vi "Serial.vi"(2 "PortName":string, 12 "Run":bool, 14 "Calibration":bool) -> (0 "DS18b20":string, 4 "DS18b20":dbl[unit][](array[numeric]), 5 "SHT11":string, 6 "MPX":dbl[](array[numeric]), 7 "MPXV7002":string, 8 "EEP":dbl[](array[numeric]), 9 "EEP":string, 10 "SHT/H":dbl[unit][](array[numeric]), 11 "Complete":bool, 15 "SHT/T":dbl[](array[numeric]))   [LabVIEW 2018]
panel:
  out "eep":bool
  out "mpxv":bool
  out "sht":bool
  out "ds":bool
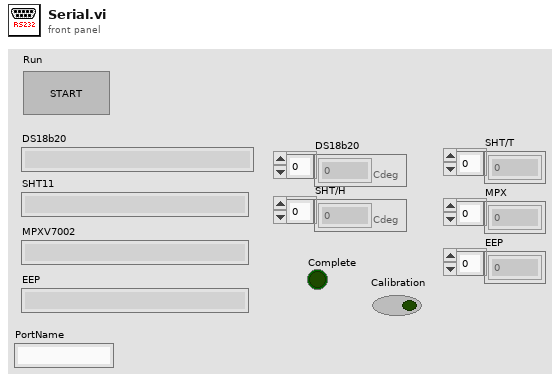
[diagram p1: front panel]
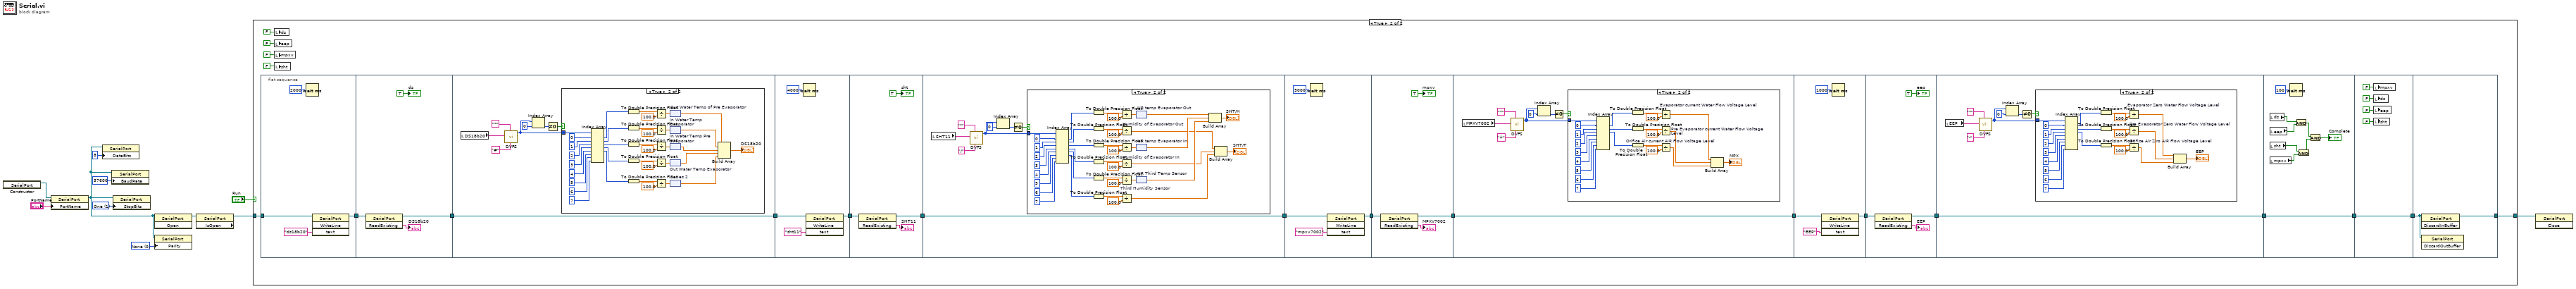
[diagram p0: block diagram]
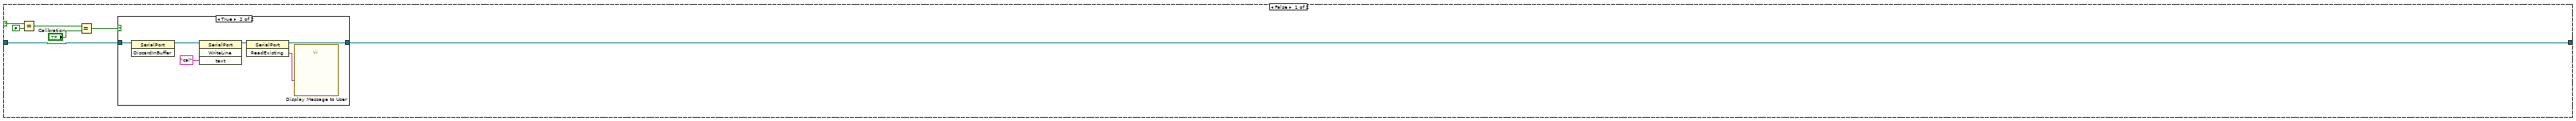
[diagram p2: hidden frame]
diagram:
  w7 = 1 items=["None", "One", "Two", "OnePointFive"] ("StopBits")
  w6 = 0 items=["None", "Odd", "Even", "Mark", "Space"] ("Parity")
  n1 = constructor class="SerialPort"() -> (reference out=w2:refnum<k24>)  [unwired: 3 in, 2 out]
  n2 = property class="SerialPort"(reference=w2, "PortName"="PortName") -> (reference out=w4:refnum<k24>)  [unwired: 1 in, 1 out]
  n3 = property class="SerialPort"(reference=w4, "DataBits"=8) -> ()  [unwired: 1 in, 2 out]
  n4 = property class="SerialPort"(reference=w4, "BaudRate"=57600) -> ()  [unwired: 1 in, 2 out]
  n5 = property class="SerialPort"(reference=w4, "StopBits"=w7) -> ()  [unwired: 1 in, 2 out]
  n6 = invoke class="SerialPort" method="Open"(reference=w4) -> (reference out=w9:refnum<k24>)  [unwired: 2 in, 2 out]
  n7 = property class="SerialPort"(reference=w4, "Parity"=w6) -> ()  [unwired: 1 in, 2 out]
  n8 = property class="SerialPort" props=["IsOpen"](reference=w9) -> (reference out=w3:refnum<k24>)  [unwired: 1 in, 2 out]
  n9 = case shown="True" "Run" {
    selector: "Run" -> [w17 _]
    tunnel: w3 -> [w18 w28]
    tunnel: [w12 w27] -> w11
    frame False {
      n10 = Equal?(x=w17, y=FALSE) -> (x = y?=w15:bool)
      n11 = Equal?(x=w15, y="Calibration") -> (x = y?=w13:bool)
      n12 = case shown="True" w13 {
        tunnel: w18 -> [w19 w21]
        tunnel: [w19 w24] -> w12
        frame False {
        }
        frame True {
          n13 = invoke class="SerialPort" method="DiscardInBuffer"(reference=w21) -> (reference out=w20:refnum<k24>)  [unwired: 2 in, 2 out]
          n14 = invoke class="SerialPort" method="WriteLine"(reference=w20, "text"="cal" ("write buffer")) -> (reference out=w25:refnum<k24>)  [unwired: 2 in, 3 out]
          n15 = invoke class="SerialPort" method="ReadExisting"(reference=w25) -> (reference out=w24:refnum<k24>, "ReadExisting"=w22:string)  [unwired: 2 in, 1 out]
          n16 = call "Display Message to User"("Message"=w22) -> ()  [unwired: 9 in, 2 out]
        }
      }
    }
    frame True {
      n17 = flat-sequence {
        tunnel: [w47] -> w45
        tunnel: w28 -> [w46]
        tunnel: w45 -> [w53]
        tunnel: [w52] -> w44
        tunnel: w44 -> [w61]
        tunnel: [w61] -> w43
        tunnel: w43 -> [w100]
        tunnel: [w97] -> w42
        tunnel: w42 -> [w103]
        tunnel: [w102] -> w41
        tunnel: w41 -> [w112]
        tunnel: [w112] -> w40
        tunnel: w40 -> [w152]
        tunnel: [w151] -> w39
        tunnel: w39 -> [w158]
        tunnel: [w156] -> w38
        tunnel: w38 -> [w166]
        tunnel: [w166] -> w37
        tunnel: w37 -> [w192]
        tunnel: [w189] -> w36
        tunnel: w36 -> [w195]
        tunnel: [w194] -> w35
        tunnel: w35 -> [w204]
        tunnel: [w204] -> w34
        tunnel: [w234] -> w33
        tunnel: w34 -> [w234]
        tunnel: w33 -> [w240]
        tunnel: [w240] -> w32
        tunnel: w32 -> [w242]
        tunnel: [w241] -> w27
        frame #0 {
          n18 = Wait (ms)(milliseconds to wait=u32 2000) -> ()  [unwired: 1 out]
          n19 = invoke class="SerialPort" method="WriteLine"(reference=w46, "text"="ds18b20") -> (reference out=w47:refnum<k24>)  [unwired: 2 in, 3 out]
        }
        frame #1 {
          n20 = invoke class="SerialPort" method="ReadExisting"(reference=w53) -> (reference out=w52:refnum<k24>, "ReadExisting"=→"DS18b20":string)  [unwired: 2 in, 1 out]
          "ds" <- TRUE ("DS")
        }
        frame #2 {
          n21 = local read "DS18b20"() -> (w55:string)
          n22 = call "DVFS.vi"("Start string"="*", "string"=w55, "end string"="#") -> ("Output"=w54:i32[])  [unwired: 3 in, 2 out]
          n23 = Index Array(array=w54, index=0) -> (element=w57:i32)
          n24 = Not Equal To 0?(x=w57) -> (x != 0?=w56:bool)
          n25 = case shown="True" w56 {
            tunnel: w54 -> [_ w96]
            frame False {
            }
            frame True {
              n26 = Index Array(array=w96, index #1=0 ("index"), index #2=1 ("index"), index #3=2 ("index"), index #4=3 ("index"), index #5=4 ("index"), index #6=5 ("index"), index #7=6 ("index"), index #8=7 ("index")) -> (element #1=w72:i32, element #2=w71:i32, element #3=w70:i32, element #4=w69:i32, element #5=w68:i32)  [unwired: 3 out]
              n27 = To Double Precision Float(number=w72) -> (double precision float=w87:dbl)
              n28 = To Double Precision Float(number=w71) -> (double precision float=w83:dbl)
              n29 = To Double Precision Float(number=w70) -> (double precision float=w81:dbl)
              n30 = To Double Precision Float(number=w69) -> (double precision float=w79:dbl)
              n31 = To Double Precision Float(number=w68) -> (double precision float=w75:dbl)
              n32 = Divide(x=w87, y=100.0) -> (x/y=w85:dbl)
              n33 = Divide(x=w83, y=100.0) -> (x/y=w84:dbl)
              n34 = Divide(x=w81, y=100.0) -> (x/y=w77:dbl)
              n35 = Divide(x=w79, y=100.0) -> (x/y=w76:dbl)
              n36 = Divide(x=w75, y=100.0) -> (x/y=w73:dbl)
              n37 = node "Out Water Temp of Pre Evaporator"(w85) -> (w67:dbl[unit])
              n38 = node "In Water Temp Evaporator"(w84) -> (w66:dbl[unit])
              n39 = node "In Water Temp Pre Evaporator"(w77) -> (w65:dbl[unit])
              n40 = node "Out Water Temp Evaporator"(w76) -> (w64:dbl[unit])
              n41 = node "Series 2"(w73) -> (w63:dbl[unit])
              n42 = Build Array(w67, w66, w65, w64, w63) -> (→"DS18b20":dbl[unit][])
            }
          }
        }
        frame #3 {
          n43 = Wait (ms)(milliseconds to wait=u32 4000) -> ()  [unwired: 1 out]
          n44 = invoke class="SerialPort" method="WriteLine"(reference=w100, "text"="sht11" ("write buffer")) -> (reference out=w97:refnum<k24>)  [unwired: 2 in, 3 out]
        }
        frame #4 {
          n45 = invoke class="SerialPort" method="ReadExisting"(reference=w103) -> (reference out=w102:refnum<k24>, "ReadExisting"=→"SHT11":string)  [unwired: 2 in, 1 out]
          "sht" <- TRUE ("SHT")
        }
        frame #5 {
          n46 = local read "SHT11"() -> (w106:string)
          n47 = call "DVFS.vi"("Start string"="*", "string"=w106, "end string"="/") -> ("Output"=w105:i32[])  [unwired: 3 in, 2 out]
          n48 = Index Array(array=w105, index=0) -> (element=w108:i32)
          n49 = Not Equal To 0?(x=w108) -> (x != 0?=w107:bool)
          n50 = case shown="True" w107 {
            tunnel: w105 -> [_ w150]
            frame False {
            }
            frame True {
              n51 = Index Array(array=w150, index #1=0 ("index"), index #2=1 ("index"), index #3=2 ("index"), index #4=3 ("index"), index #5=4 ("index"), index #6=5 ("index"), index #7=6 ("index"), index #8=7 ("index")) -> (element #1=w126:i32, element #2=w125:i32, element #3=w124:i32, element #4=w123:i32, element #5=w122:i32, element #6=w121:i32)  [unwired: 2 out]
              n52 = To Double Precision Float(number=w126) -> (double precision float=w141:dbl)
              n53 = To Double Precision Float(number=w125) -> (double precision float=w132:dbl)
              n54 = To Double Precision Float(number=w124) -> (double precision float=w139:dbl)
              n55 = To Double Precision Float(number=w123) -> (double precision float=w130:dbl)
              n56 = To Double Precision Float(number=w122) -> (double precision float=w137:dbl)
              n57 = To Double Precision Float(number=w121) -> (double precision float=w128:dbl)
              n58 = Divide(x=w141, y=100.0) -> (x/y=w135:dbl)
              n59 = Divide "Humidity of Evaporator Out"(x=w132, y=100.0) -> (x/y=w117:dbl)
              n60 = Divide(x=w139, y=100.0) -> (x/y=w134:dbl)
              n61 = Divide "Humidity of Evaporator In"(x=w130, y=100.0) -> (x/y=w116:dbl)
              n62 = Divide(x=w137, y=100.0) -> (x/y=w133:dbl)
              n63 = Divide "Third Humidity Sensor"(x=w128, y=100.0) -> (x/y=w115:dbl)
              n64 = node "AIR temp Evaporator Out"(w135) -> (w120:dbl[unit])
              n65 = node "AIR temp Evaporator In"(w134) -> (w119:dbl[unit])
              n66 = node "AIR Third Temp Sensor"(w133) -> (w118:dbl[unit])
              n67 = Build Array(w120, w119, w118) -> (→"SHT/H":dbl[unit][])
              n68 = Build Array(w117, w116, w115) -> (→"SHT/T":dbl[])
            }
          }
        }
        frame #6 {
          n69 = Wait (ms)(milliseconds to wait=u32 5000) -> ()  [unwired: 1 out]
          n70 = invoke class="SerialPort" method="WriteLine"(reference=w152, "text"="mpxv7002" ("write buffer")) -> (reference out=w151:refnum<k24>)  [unwired: 2 in, 3 out]
        }
        frame #7 {
          n71 = invoke class="SerialPort" method="ReadExisting"(reference=w158) -> (reference out=w156:refnum<k24>, "ReadExisting"=→"MPXV7002":string)  [unwired: 2 in, 1 out]
          "mpxv" <- TRUE ("MPXV")
        }
        frame #8 {
          n72 = local read "MPXV7002"() -> (w160:string)
          n73 = call "DVFS.vi"("Start string"="*", "string"=w160, "end string"="+") -> ("Output"=w159:i32[])  [unwired: 3 in, 2 out]
          n74 = Index Array(array=w159, index=0) -> (element=w162:i32)
          n75 = Not Equal To 0?(x=w162) -> (x != 0?=w161:bool)
          n76 = case shown="True" w161 {
            tunnel: w159 -> [_ w188]
            frame False {
            }
            frame True {
              n77 = Index Array(array=w188, index #1=0 ("index"), index #2=1 ("index"), index #3=2 ("index"), index #4=3 ("index"), index #5=4 ("index"), index #6=5 ("index"), index #7=6 ("index"), index #8=7 ("index")) -> (element #1=w173:i32, element #2=w172:i32, element #3=w171:i32)  [unwired: 5 out]
              n78 = To Double Precision Float(number=w173) -> (double precision float=w179:dbl)
              n79 = To Double Precision Float(number=w172) -> (double precision float=w177:dbl)
              n80 = To Double Precision Float(number=w171) -> (double precision float=w175:dbl)
              n81 = Divide "Evaporator current Water Flow Voltage Level"(x=w179, y=100.0) -> (x/y=w170:dbl)
              n82 = Divide "Pre Evaporator current Water Flow Voltage Level"(x=w177, y=100.0) -> (x/y=w169:dbl)
              n83 = Divide "Orifice Air current AIR Flow Voltage Level"(x=w175, y=100.0) -> (x/y=w168:dbl)
              n84 = Build Array(w170, w169, w168) -> (→"MPX":dbl[])
            }
          }
        }
        frame #9 {
          n85 = invoke class="SerialPort" method="WriteLine"(reference=w192, "text"="EEP" ("write buffer")) -> (reference out=w189:refnum<k24>)  [unwired: 2 in, 3 out]
          n86 = Wait (ms)(milliseconds to wait=u32 1000) -> ()  [unwired: 1 out]
        }
        frame #10 {
          n87 = invoke class="SerialPort" method="ReadExisting"(reference=w195) -> (reference out=w194:refnum<k24>, "ReadExisting"=→"EEP":string)  [unwired: 2 in, 1 out]
          "eep" <- TRUE ("EEP")
        }
        frame #11 {
          n88 = local read "EEP"() -> (w198:string)
          n89 = call "DVFS.vi"("Start string"="*", "string"=w198, "end string"="-") -> ("Output"=w197:i32[])  [unwired: 3 in, 2 out]
          n90 = Index Array(array=w197, index=0) -> (element=w200:i32)
          n91 = Not Equal To 0?(x=w200) -> (x != 0?=w199:bool)
          n92 = case shown="True" w199 {
            tunnel: w197 -> [_ w226]
            frame False {
            }
            frame True {
              n93 = Index Array(array=w226, index #1=0 ("index"), index #2=1 ("index"), index #3=2 ("index"), index #4=3 ("index"), index #5=4 ("index"), index #6=5 ("index"), index #7=6 ("index"), index #8=7 ("index")) -> (element #1=w211:i32, element #2=w209:i32, element #3=w210:i32)  [unwired: 5 out]
              n94 = To Double Precision Float(number=w211) -> (double precision float=w217:dbl)
              n95 = To Double Precision Float(number=w209) -> (double precision float=w215:dbl)
              n96 = To Double Precision Float(number=w210) -> (double precision float=w213:dbl)
              n97 = Divide "Evaporator Zero Water Flow Voltage Level"(x=w217, y=100.0) -> (x/y=w208:dbl)
              n98 = Divide "Pre Evaporator Zero Water Flow Voltage Level"(x=w215, y=100.0) -> (x/y=w207:dbl)
              n99 = Divide "Orifice Air Ziro AIR Flow Voltage Level"(x=w213, y=100.0) -> (x/y=w206:dbl)
              n100 = Build Array(w208, w207, w206) -> (→"EEP":dbl[])
            }
          }
        }
        frame #12 {
          n101 = local read "ds"() -> (w233:bool)
          n102 = local read "eep"() -> (w232:bool)
          n103 = local read "sht"() -> (w230:bool)
          n104 = local read "mpxv"() -> (w231:bool)
          n105 = Wait (ms)(milliseconds to wait=u32 100) -> ()  [unwired: 1 out]
          n106 = And(x=w233, y=w232) -> (x .and. y?=w228:bool)
          n107 = And(x=w230, y=w231) -> (x .and. y?=w229:bool)
          n108 = And(x=w228, y=w229) -> (x .and. y?=→"Complete":bool)
        }
        frame #13 {
          n109 = local write "mpxv"(FALSE ("mpxv")) -> ()
          n110 = local write "ds"(FALSE ("eep")) -> ()
          n111 = local write "eep"(FALSE ("DS")) -> ()
          n112 = local write "sht"(FALSE ("sht")) -> ()
        }
        frame #14 {
          n113 = invoke class="SerialPort" method="DiscardInBuffer"(reference=w242) -> (reference out=w241:refnum<k24>)  [unwired: 2 in, 2 out]
          n114 = invoke class="SerialPort" method="DiscardOutBuffer"(reference=w242) -> ()  [unwired: 2 in, 3 out]
        }
      }
      n115 = local write "ds"(FALSE ("DS")) -> ()
      n116 = local write "eep"(FALSE ("eep")) -> ()
      n117 = local write "mpxv"(FALSE ("mpxv")) -> ()
      n118 = local write "sht"(FALSE ("sht")) -> ()
    }
  }
  n119 = invoke class="SerialPort" method="Close"(reference=w11) -> ()  [unwired: 2 in, 3 out]
